vi "_Raise Content Loading.vi"(4 "WebView2.lvlib:WebView2 Control.lvclass":refnum<class "WebView2 Control.lvclass">, 5 "Event Data":cluster{"sender":refnum<k24>, "e":refnum<k24>}, 6 "Control Ref":refnum<k24>, 7 "Event Common Data":T1) -> ()   [LabVIEW 2025, in "WebView2.lvlib" / "WebView2 Control.lvclass"]
uses:
  WebView2 Control.lvclass
  WebView2 Control.lvclass/WebView2 Control.ctl
  E:/Labview/LV 2023/PPL/PPL Builder/Libs/LV-WebView2/Source/Libs/Microsoft.Web.WebView2.Core.dll
  Libs/Microsoft.Web.WebView2.Core.dll
  Content Loading Event Data.ctl
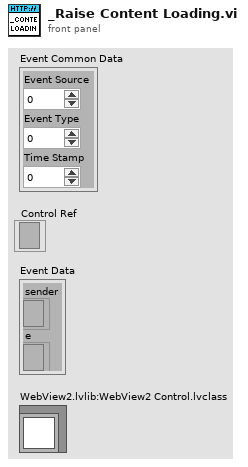
[diagram p1: front panel]
types:
  T1 = cluster{"Event Source":i32, "Event Type":u32, "Time Stamp":u32}
  T2 = typedef "WebView2.lvlib/WebView2 Control.lvclass/Content Loading Event Data.ctl" = cluster{"IsErrorPage":bool, "NavigationId":u64}
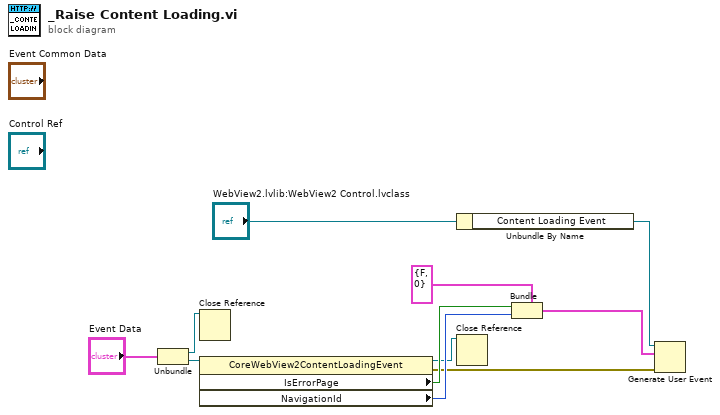
[diagram p0: block diagram]
diagram:
  n1 = Unbundle("Event Data") -> ("sender"=w10:refnum<k24>, "e"=w9:refnum<k24>)
  n2 = Close Reference(reference=w10) -> ()  [unwired: 1 in, 1 out]
  n3 = property class="CoreWebView2ContentLoadingEvent"(reference=w9) -> (reference out=w1:refnum<k24>, error out=w2:errorcluster, "IsErrorPage"=w8:bool, "NavigationId"=w7:u64)  [unwired: 1 in]
  n4 = Unbundle By Name("WebView2.lvlib:WebView2 Control.lvclass") -> ("Content Loading Event"=w4:refnum<user-event>)
  n5 = Close Reference(reference=w1) -> ()  [unwired: 1 in, 1 out]
  n6 = Bundle(cluster=T2 {"IsErrorPage"=FALSE, "NavigationId"=0}, "IsErrorPage"=w8, "NavigationId"=w7) -> (w3:T2)
  n7 = Generate User Event(user event=w4, event data cluster=w3, error in=w2) -> ()  [unwired: 1 in, 2 out]
